vi "Stop Core.vi"(10 "final error code":i32, 11 "Gage digitizer actor in":refnum<class "Gage digitizer actor.lvclass">) -> (3 "Gage digitizer actor out":refnum<class "Gage digitizer actor.lvclass">)   [LabVIEW 2015, in "Gage digitizer actor.lvclass"]
doc: "(<B>Filename</B>: Actor Framework.lvlib:Actor.lvclass:Stop Core.vi)\n\nDefines what the actor does before it stops. Use the <B>final error code</B> input to determine whether the actor shut down in response to an error.\n\nBy default, this method does nothing. A descendant class may override it to define behavior, such as shutting down any processes the actor initiated in its override of the Actor Core method."
uses:
  Gage digitizer actor.lvclass
  Gage digitizer actor.lvclass/Gage digitizer actor.ctl
  <vilib>/ActorFramework/Actor/Actor.lvclass
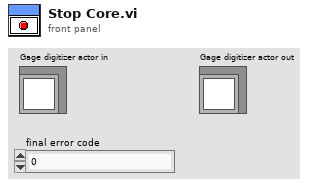
[diagram p1: front panel]
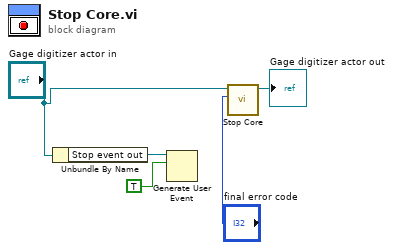
[diagram p0: block diagram]
diagram:
  n1 = Unbundle By Name("Gage digitizer actor in") -> ("Stop event out"=w2:refnum<user-event>)
  n2 = Generate User Event(user event=w2, event data cluster=TRUE ("event data")) -> ()  [unwired: 2 in, 2 out]
  n3 = call-parent "Stop Core.vi"("final error code"="final error code", "Actor in"="Gage digitizer actor in") -> ("Actor out"=→"Gage digitizer actor out":refnum<class "Gage digitizer actor.lvclass">)  [unwired: 9 in]
